vi "tiffReader-small_file_read-DSJ.vi"(4 "error in":errorcluster, 5 "Flip Width/Length?":bool, 6 "Data in IFD\n(small files)":bool, 7 "File Path":path) -> (0 "error out":errorcluster, 1 "frames loaded":i32, 2 "Array 3":u16[][][](array[numeric]), 3 "width":i32)   [LabVIEW 2012]
panel:
  out "error out 2":errorcluster
  out "Data":u16[][](graph)
  out "2D array":u16[][](graph)
  out "bits/sample":i32
  out "length":i32
  out "offset/values":i32[](array[numeric]) format="%0d"
  out "counts":i32[](array[numeric])
  out "types":i16[](array[numeric])
  out "field tags":i16[](array[numeric])
  out "ifd entry count":i16
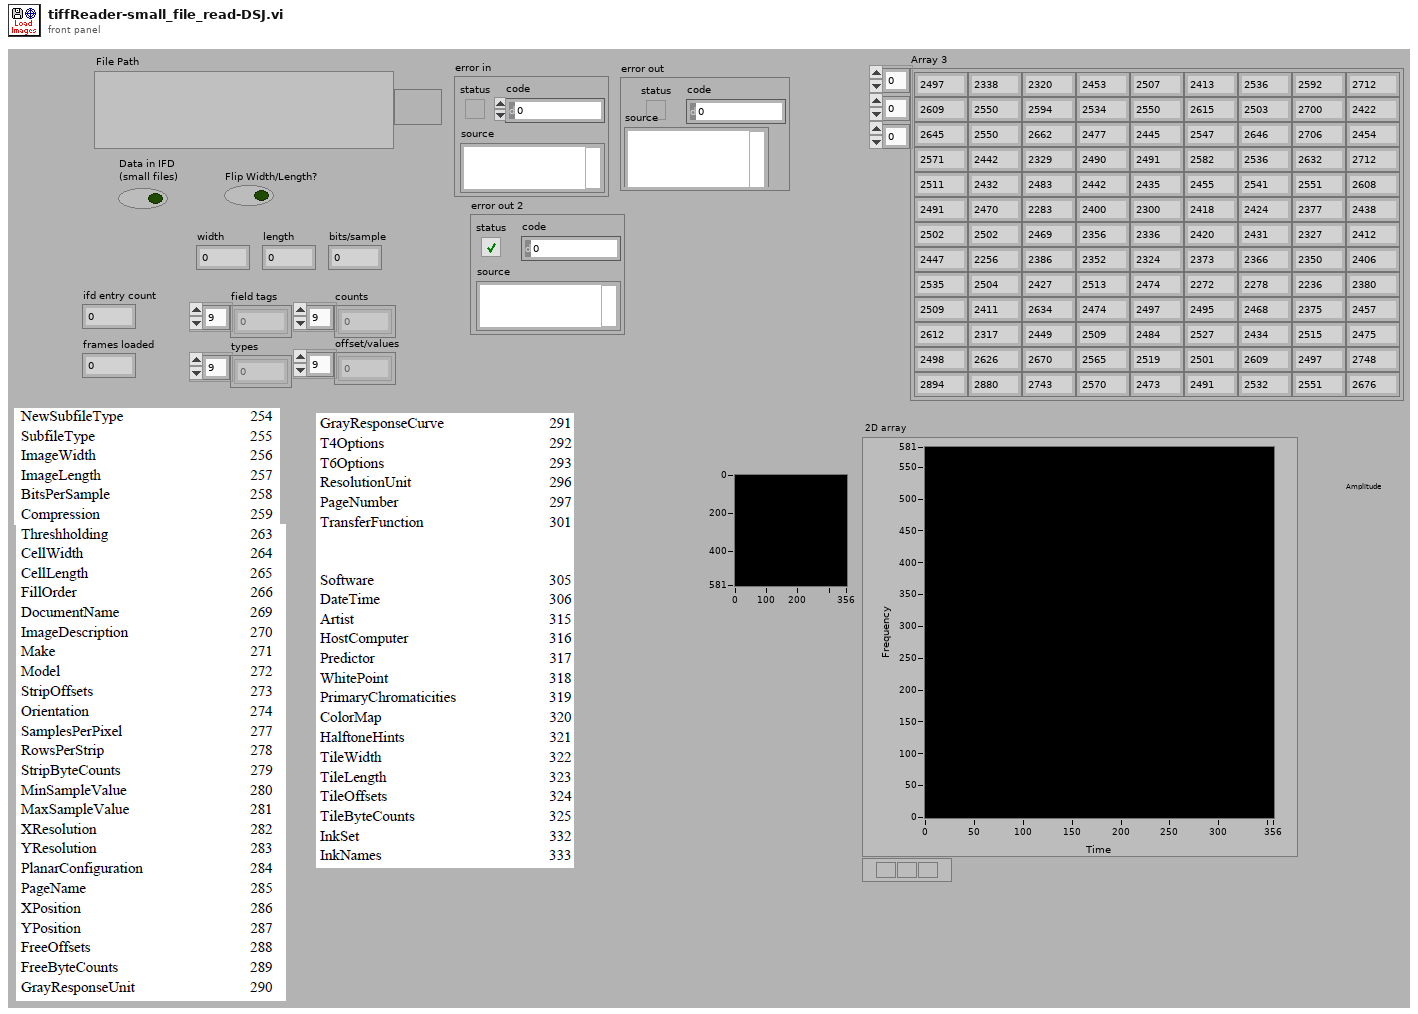
[diagram p1: front panel]
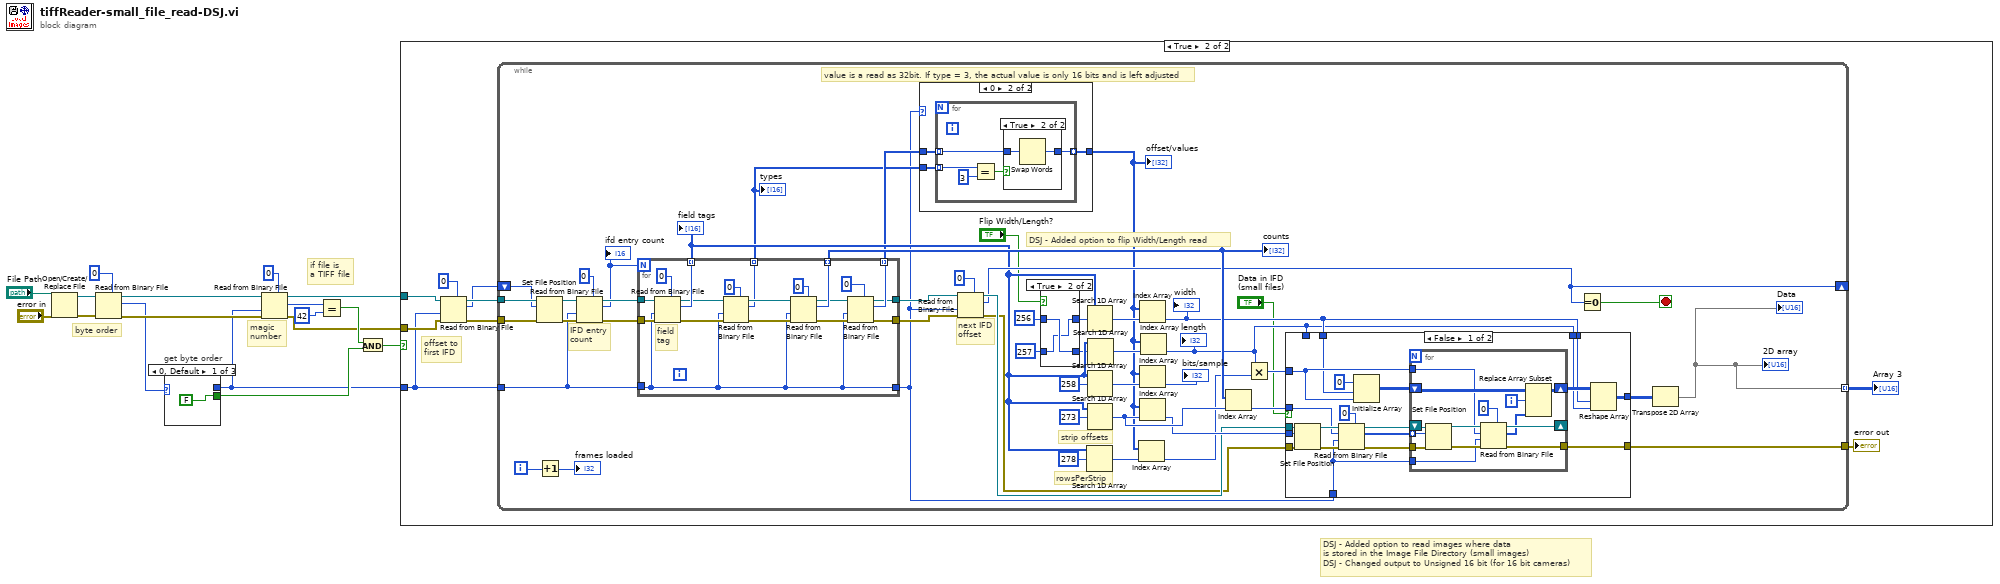
[diagram p0: block diagram]
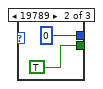
[diagram p2: hidden frame]
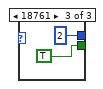
[diagram p3: hidden frame]
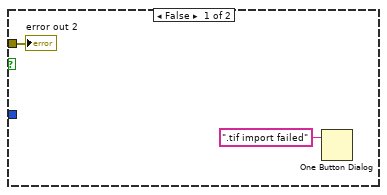
[diagram p4: hidden frame]
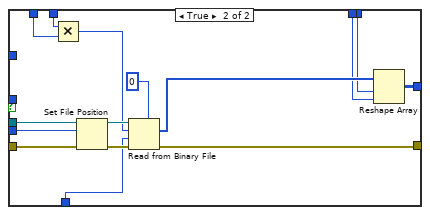
[diagram p5: hidden frame]
diagram:
  # "DSJ - Added option to read images where data\nis stored in the Image File Directory (small images)\nDSJ - Changed output to Unsigned 16 bit (for 16 bit cameras)"
  # "if file is\na TIFF file"
  # "magic\nnumber"
  # "byte order"
  n1 = Open/Create/Replace File(file path (use dialog)="File Path", error in="error in") -> (refnum out=w16:refnum<file>, error out=w17:errorcluster)  [unwired: 4 in, 1 out]
  n2 = Read from Binary File(5:i16 0, 8:w17, 11:w16) -> (0:w12:errorcluster, 2:w5:i16, 3:w14:refnum<file>)  [unwired: 3 in, 1 out]
  n3 = case "get byte order" shown="0, Default" w5 {
    tunnel: [_ 0 2] -> w2
    tunnel: [FALSE TRUE TRUE] -> w4
    frame 0, Default {
    }
    frame 19789 {
    }
    frame 18761 {
    }
  }
  n4 = Read from Binary File(5:i16 0, 8:w12, 9:w2, 11:w14) -> (0:w6:errorcluster, 2:w11:i16, 3:w7:refnum<file>)  [unwired: 2 in, 1 out]
  n5 = Equal?(x=w11, y=i16 42) -> (x = y?=w9:bool)
  n6 = And(x=w9, y=w4) -> (x .and. y?=w8:bool)
  n7 = case shown="True" w8 {
    tunnel: w7 -> [_ w33]
    tunnel: w6 -> [w23 w32]
    tunnel: w2 -> [_ w28]
    frame False {
      n8 = One Button Dialog(message=".tif import failed") -> ()  [unwired: 1 in, 1 out]
      "error out 2" <- w23
    }
    frame True {
      # "offset to\nfirst IFD"
      n9 = Read from Binary File(5:0, 8:w32, 9:w28, 11:w33) -> (0:w30:errorcluster, 2:w27:i32, 3:w29:refnum<file>)  [unwired: 2 in, 1 out]
      n10 = while {
        tunnel: w30 -> [w82]
        tunnel: w29 -> [w81]
        tunnel: w28 -> [w59]
        shift-right: [w61] -> _
        shift-left: w27 -> [w62]
        tunnel: [w34] -> w25 mode=indexing
        tunnel: [w51] -> w26
        i -> [w37]
        stop <- w60 stop-if-true
        # "DSJ - Added option to flip Width/Length read"
        # "value is a read as 32bit. If type = 3, the actual value is only 16 bits and is left adjusted"
        # "rowsPerStrip"
        # "strip offsets"
        # "next IFD\noffset"
        # "IFD entry\ncount"
        n11 = Set File Position(offset (in bytes) (0)=w62, refnum=w81, error in=w82) -> (refnum out=w79:refnum<file>, error out=w78:errorcluster)  [unwired: 1 in]
        n12 = Increment(x=w37) -> (x+1=→"frames loaded":i32)
        n13 = Read from Binary File(5:i16 0, 8:w78, 9:w59, 11:w79) -> (0:w76:errorcluster, 2:w75:i16, 3:w77:refnum<file>)  [unwired: 2 in, 1 out]
        "ifd entry count" <- w75
        n14 = for {
          N: w75 -> [_]
          tunnel: w77 -> [w165]
          tunnel: w76 -> [w164]
          tunnel: [w163] -> w49 mode=indexing
          tunnel: [w151] -> w47 mode=indexing
          tunnel: [w157] -> w68 mode=indexing
          tunnel: [w153] -> w48 mode=indexing
          tunnel: w59 -> [w149]
          tunnel: [w152] -> w65
          tunnel: [w149] -> w41
          tunnel: [w148] -> w53
          # "field\ntag"
          n15 = Read from Binary File(5:i16 0, 8:w164, 9:w149, 11:w165) -> (0:w161:errorcluster, 2:w163:i16, 3:w162:refnum<file>)  [unwired: 2 in, 1 out]
          n16 = Read from Binary File(5:i16 0, 8:w161, 9:w149, 11:w162) -> (0:w156:errorcluster, 2:w151:i16, 3:w158:refnum<file>)  [unwired: 2 in, 1 out]
          n17 = Read from Binary File(5:0, 8:w156, 9:w149, 11:w158) -> (0:w155:errorcluster, 2:w157:i32, 3:w154:refnum<file>)  [unwired: 2 in, 1 out]
          n18 = Read from Binary File(5:0, 8:w155, 9:w149, 11:w154) -> (0:w148:errorcluster, 2:w153:i32, 3:w152:refnum<file>)  [unwired: 2 in, 1 out]
        }
        "field tags" <- w49
        "types" <- w47
        "counts" <- w68
        n19 = case shown="0" w41 {
          tunnel: [w136 w137] -> w50
          tunnel: w48 -> [w136 w139]
          tunnel: w47 -> [_ w138]
          frame 2, Default {
          }
          frame 0 {
            n20 = for {
              tunnel: w138 -> [w143] mode=indexing
              tunnel: w139 -> [w141] mode=indexing
              tunnel: [w140] -> w137 mode=indexing
              n21 = Equal?(x=w143, y=3) -> (x = y?=w142:bool)
              n22 = case shown="True" w142 {
                tunnel: w141 -> [w145 w147]
                tunnel: [w145 w146] -> w140
                frame False {
                }
                frame True {
                  n23 = Swap Words(1:w147) -> (0:w146:i32)
                }
              }
            }
          }
        }
        "offset/values" <- w50
        n24 = Read from Binary File(5:0, 8:w53, 9:w41, 11:w65) -> (0:w52:errorcluster, 2:w61:i32, 3:w63:refnum<file>)  [unwired: 2 in, 1 out]
        n25 = case shown="True" "Flip Width/Length?" {
          tunnel: [w132 w134] -> w46
          tunnel: [w133 w135] -> w45
          tunnel: i16 257 ("element") -> [w133 w134]
          tunnel: i16 256 ("element") -> [w132 w135]
          frame False {
          }
          frame True {
          }
        }
        n26 = Search 1D Array(1D array=w49, element=i16 278) -> (index of element=w56:i32)  [unwired: 1 in]
        n27 = Search 1D Array(1D array=w49, element=w46) -> (index of element=w74:i32)  [unwired: 1 in]
        n28 = Search 1D Array(1D array=w49, element=i16 258) -> (index of element=w71:i32)  [unwired: 1 in]
        n29 = Search 1D Array(1D array=w49, element=i16 273) -> (index of element=w67:i32)  [unwired: 1 in]
        n30 = Search 1D Array(1D array=w49, element=w45) -> (index of element=w73:i32)  [unwired: 1 in]
        n31 = Index Array(array=w50, index=w56) -> (element=w55:i32)
        n32 = Index Array(array=w50, index=w74) -> (element=w40:i32)
        "width" <- w40
        n33 = Index Array(array=w50, index=w71) -> (element=→"bits/sample":i32)
        n34 = Index Array(array=w50, index=w67) -> (element=w66:i32)
        n35 = Index Array(array=w50, index=w73) -> (element=w39:i32)
        "length" <- w39
        n36 = Index Array(array=w68, index=w67) -> (element=w58:i32)
        n37 = Multiply(x=w39, y=w55) -> (x*y=w54:i32)
        n38 = case shown="False" "Data in IFD\n(small files)" {
          tunnel: w66 -> [w95 w127]
          tunnel: w63 -> [w94 w129]
          tunnel: w58 -> [w93 _]
          tunnel: w54 -> [w92 _]
          tunnel: w40 -> [w91 w126]
          tunnel: w52 -> [w90 w128]
          tunnel: [w89 w124] -> w51
          tunnel: w41 -> [w88 w119]
          tunnel: w39 -> [_ w125]
          tunnel: [w84 w118] -> w35
          tunnel: w40 -> [w86 w121]
          tunnel: w39 -> [w85 w120]
          frame False {
            n39 = Set File Position(offset (in bytes) (0)=w95, refnum=w94, error in=w90) -> (refnum out=w102:refnum<file>, error out=w101:errorcluster)  [unwired: 1 in]
            n40 = Read from Binary File(5:0, 8:w101, 9:w88, 10:w93, 11:w102) -> (0:w97:errorcluster, 2:w99:i32[], 3:w98:refnum<file>)  [unwired: 1 in, 1 out]
            n41 = Initialize Array(u16 0, w91, w92) -> (w96:u16[][])
            n42 = for {
              tunnel: w99 -> [w116] mode=indexing
              tunnel: w97 -> [w114]
              tunnel: w88 -> [w111]
              shift-right: [w108] -> w87
              shift-left: w96 -> [w110]
              shift-right: [w107] -> _
              shift-left: w98 -> [w115]
              tunnel: w92 -> [w105]
              tunnel: [w104] -> w89
              i -> [w109]
              n43 = Set File Position(offset (in bytes) (0)=w116, refnum=w115, error in=w114) -> (refnum out=w113:refnum<file>, error out=w112:errorcluster)  [unwired: 1 in]
              n44 = Read from Binary File(5:u16 0, 8:w112, 9:w111, 10:w105, 11:w113) -> (0:w104:errorcluster, 2:w106:u16[], 3:w107:refnum<file>)  [unwired: 1 in, 1 out]
              n45 = Replace Array Subset(array=w110, new element=w106, index (row)=w109) -> (w108:u16[][])  [unwired: 1 in]
            }
            n46 = Reshape Array(w87, w86, w85) -> (w84:u16[][])
          }
          frame True {
            n47 = Multiply(x=w126, y=w125) -> (x*y=w123:i32)
            n48 = Set File Position(offset (in bytes) (0)=w127, refnum=w129, error in=w128) -> (refnum out=w131:refnum<file>, error out=w130:errorcluster)  [unwired: 1 in]
            n49 = Read from Binary File(5:u16 0, 8:w130, 9:w119, 10:w123, 11:w131) -> (0:w124:errorcluster, 2:w122:u16[])  [unwired: 1 in, 2 out]
            n50 = Reshape Array(w122, w121, w120) -> (w118:u16[][])
          }
        }
        n51 = Equal To 0?(x=w61) -> (x = 0?=w60:bool)
        n52 = Transpose 2D Array(2D array=w35) -> (transposed array=w34:u16[][])
        "2D array" <- w34
        "Data" <- w34
      }
      "error out" <- w26
      "Array 3" <- w25
    }
  }
